vi "Write Atts.vi"(6 "Points":i32, 7 "IF_Band":dbl, 8 "error in (no error)":errorcluster, 9 "Stop":dbl, 10 "Start":dbl, 11 "RS in":refnum<class "RS.lvclass">) -> (0 "error out":errorcluster, 3 "RS out":refnum<class "RS.lvclass">)   [LabVIEW 2015, in "RS.lvclass"]
uses:
  RS.lvclass
  RS.lvclass/RS.ctl
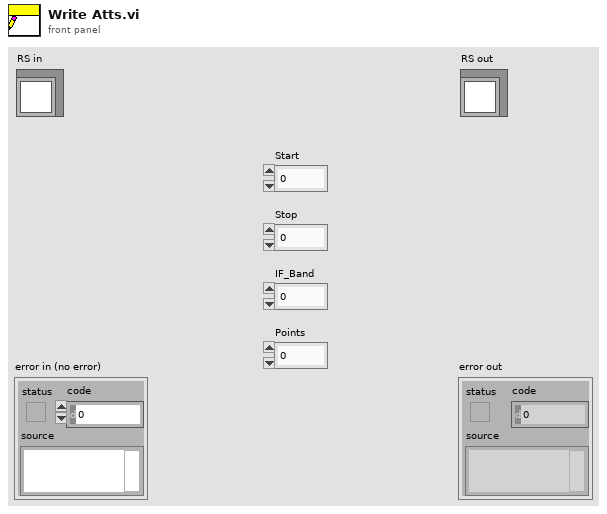
[diagram p1: front panel]
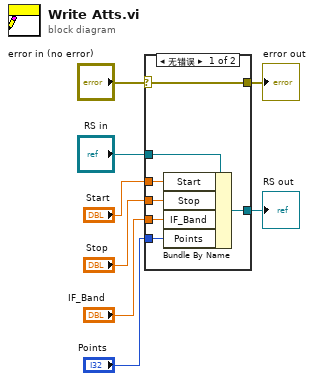
[diagram p0: block diagram]
diagram:
  n1 = case shown="无错误" "error in (no error)" {
    selector: "error in (no error)" -> [w15 w16]
    tunnel: [w15 w16] -> w5
    tunnel: [w13 w17] -> w7
    tunnel: "RS in" -> [w14 w17]
    tunnel: "Start" -> [w12 _]
    tunnel: "Points" -> [w11 _]
    tunnel: "IF_Band" -> [w10 _]
    tunnel: "Stop" -> [w9 _]
    frame No Error {
      n2 = Bundle By Name(cluster=w14, "Start"=w12, "Stop"=w9, "IF_Band"=w10, "Points"=w11) -> (w13:refnum<class "RS.lvclass">)
    }
    frame Error {
    }
  }
  "error out" <- w5
  "RS out" <- w7
